vi "Power Start Trigger.vi"(8 "error in (no error)":errorcluster, 10 "Number of samples":i64, 11 "IVI Refnum in":refnum<k15>) -> (0 "error out":errorcluster, 2 "data":cdb[](array[numeric]), 3 "IVI Refnum out":refnum<k15>)   [LabVIEW 2012]
uses:
  <instrlib>/niUSRP/niUSRP Fetch Rx Data (CDB).vi
panel:
  in  "Trigger Level":dbl
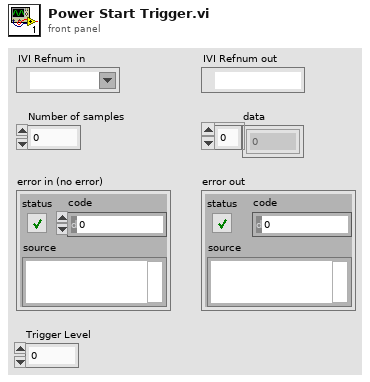
[diagram p1: front panel]
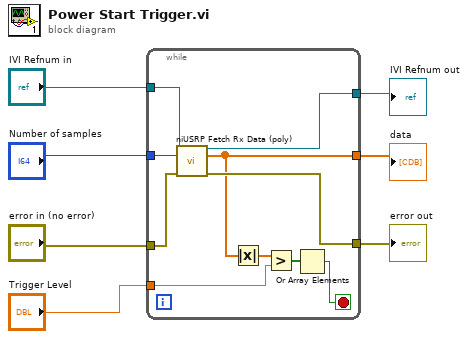
[diagram p0: block diagram]
diagram:
  n1 = while {
    tunnel: [w11] -> w7
    tunnel: [w17] -> w6
    tunnel: [w16] -> w5
    tunnel: "error in (no error)" -> [w15]
    tunnel: "Number of samples" -> [w14]
    tunnel: "IVI Refnum in" -> [w13]
    tunnel: "Trigger Level" -> [w10]
    stop <- w8 stop-if-true
    n2 = call-poly <instrlib>:"niUSRP Fetch Rx Data (poly).vi"("session handle"=w13, "number of samples"=w14, "error in (no error)"=w15) -> ("session handle out"=w17:refnum<k15>, "data"=w11:cdb[], "error out"=w16:errorcluster)  [unwired: 9 in, 1 out]
    n3 = Absolute Value(x=w11) -> (abs(x)=w12:dbl[])
    n4 = Greater?(x=w12, y=w10) -> (0:w9:bool[])
    n5 = Or Array Elements(Boolean array=w9) -> (logical OR=w8:bool)
  }
  "data" <- w7
  "IVI Refnum out" <- w6
  "error out" <- w5
